vi "compare if zero.vi"(5 "if zero out":dbl=1.1 format="%#_13g", 6 "Numeric":dbl format="%#_13g") -> (2 "out":dbl)   [LabVIEW 2016]
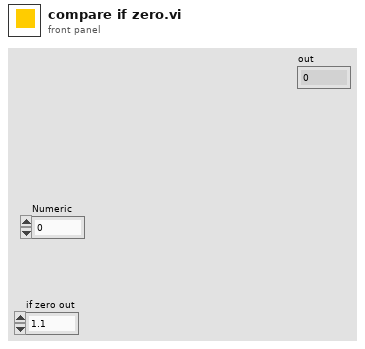
[diagram p1: front panel]
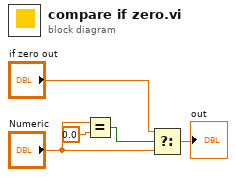
[diagram p0: block diagram]
diagram:
  n1 = Equal?(x="Numeric", y=0.0) -> (x = y?=w4:bool)
  n2 = Select(t="if zero out", s=w4, f="Numeric") -> (s? t:f=→"out":dbl)
